vi "Variant Dictionary to JSON String.vi"(8 "error in (no error)":errorcluster, 11 "Registry In":variant) -> (0 "error out":errorcluster, 3 "JSON String":string)   [LabVIEW 2018, in "ClientMessaging.lvlib"]
uses:
  ClientMessaging.lvlib
  <vilib>/JDP Science/JSONtext/JSONtext.lvlib
panel:
  in  "Select Keys Regexp":string=".*"
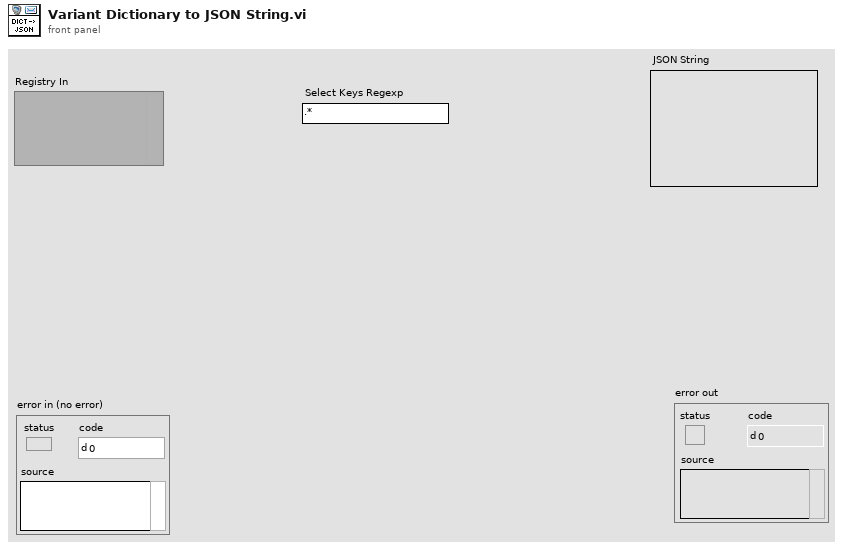
[diagram p1: front panel]
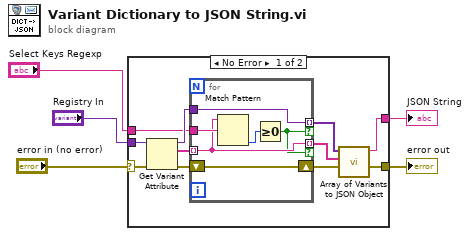
[diagram p0: block diagram]
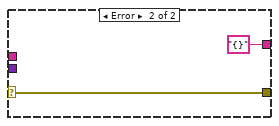
[diagram p2: hidden frame]
diagram:
  n1 = case shown="No Error" "error in (no error)" {
    selector: "error in (no error)" -> [w15 w24]
    tunnel: "Registry In" -> [w16 _]
    tunnel: "Select Keys Regexp" -> [w12 _]
    tunnel: [w6 w24] -> w2
    tunnel: [w7 "{}" ("<JSON>")] -> w1
    frame No Error {
      n2 = Get Variant Attribute(Variant=w16, error in=w15) -> (duplicate Variant=w14:variant, names=w13:string[], error out=w11:errorcluster)  [unwired: 2 in, 1 out]
      n3 = for {
        tunnel: w14 -> [w19]
        tunnel: w13 -> [w18] mode=indexing
        tunnel: w12 -> [w22]
        shift-right: [w21] -> w10
        shift-left: w11 -> [w21]
        tunnel: [w19] -> w8 mode=indexing if=w17
        tunnel: [w18] -> w9 mode=indexing if=w17
        n4 = Match Pattern(string=w18, regular expression=w22) -> (offset past match=w20:i32)  [unwired: 1 in, 3 out]
        n5 = Greater Or Equal To 0?(x=w20) -> (x >= 0?=w17:bool)
      }
      n6 = call <vilib>:"Array of Variants to JSON Object.vi"("error in (no error)"=w10, "Names"=w9, "Array"=w8) -> ("error out"=w6:errorcluster, "<JSON>"=w7:string)  [unwired: 7 in]
    }
    frame Error {
    }
  }
  "error out" <- w2
  "JSON String" <- w1
